vi "client.vi"() -> ()   [LabVIEW 2016]
uses:
  defs/Control 1.ctl
  defs/Control 3.ctl
  defs/Control 2.ctl
  defs/Control 6.ctl
  defs/Control 5.ctl
  defs/Control 4.ctl
panel:
  in  "czestotl [Hz]":T1=1.0
  in  "jaki sygna³?":T2 items=["sin", "square", "sawtooth", "noise"]
  in  "z jakim?":T3 items=["sin", "square", "sawtooth", "noise"]
  in  "dzialanie":T4 items=["+", "-", "*", "/", ""]
  in  "amplituda":T5=10.0 caption="Frequency"
  in  "x pocz":T1
  in  "Clear":bool
  out "wynik dzialania":cluster{"Y":dbl[], "Y":dbl[]}[](graph)
  in  "krok [ms]":T6=50.0 caption="Frequency"
  in  "Stop":bool
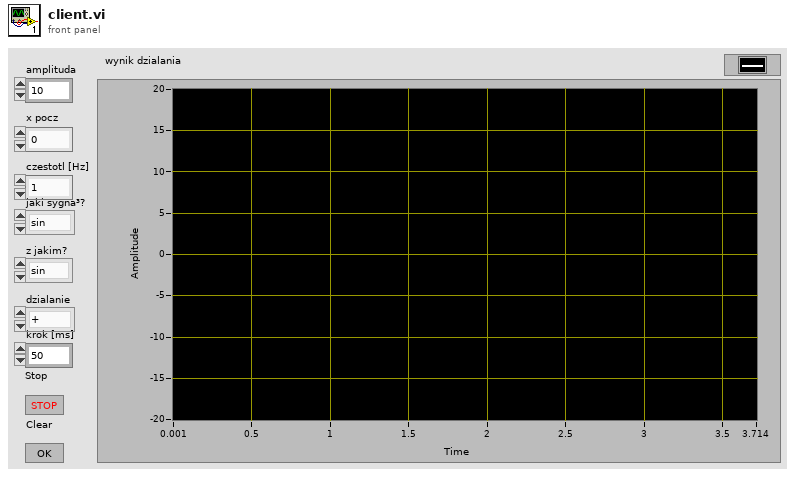
[diagram p1: front panel]
types:
  T1 = typedef "Control 3.ctl" = dbl
  T2 = typedef "Control 4.ctl" = u16
  T3 = typedef "Control 5.ctl" = u16
  T4 = typedef "Control 6.ctl" = u16
  T5 = typedef "Control 2.ctl" = dbl
  T6 = typedef "Control 1.ctl" = dbl
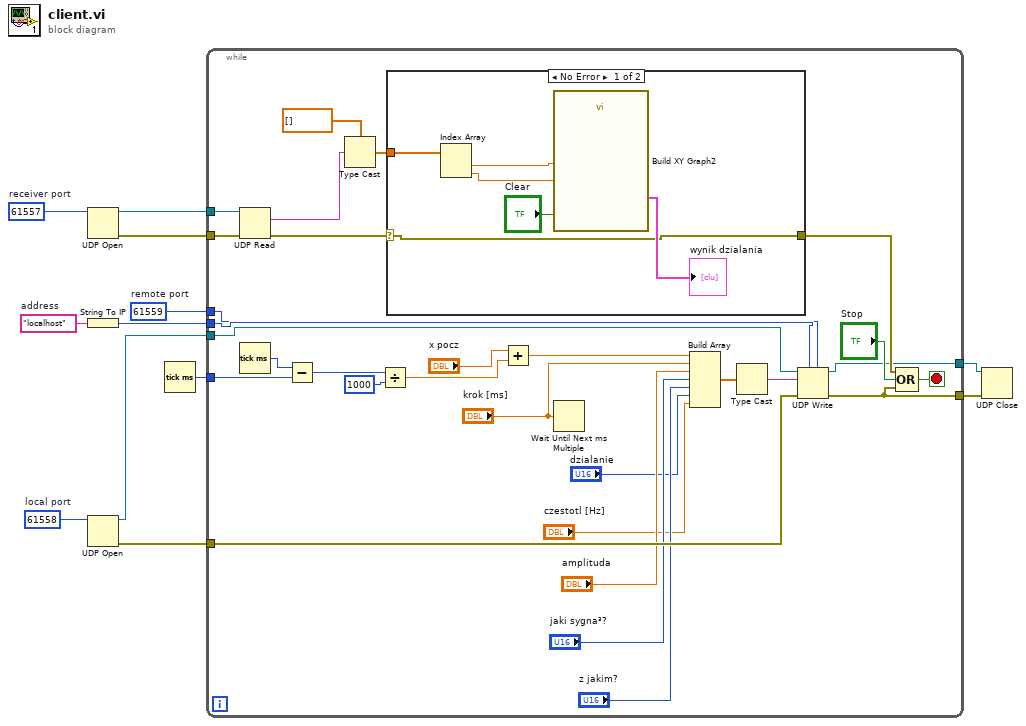
[diagram p0: block diagram]
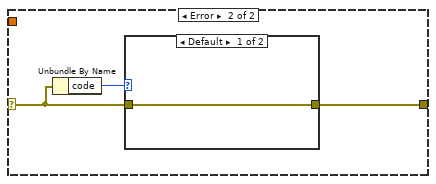
[diagram p2: hidden frame]
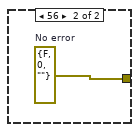
[diagram p3: hidden frame]
diagram:
  w3 = u16 61559  # remote port
  w8 = u16 61558  # local port
  w9 = "localhost"  # address
  w12 = u16 61557  # receiver port
  n1 = UDP Open(11:w12) -> (port=w11:refnum<k16>, 0:w10:errorcluster)  [unwired: 4 in, 1 out]
  n2 = String To IP(1:w9) -> (0:w6:u32)
  n3 = UDP Open(11:w8) -> (port=w4:refnum<k16>, 0:w5:errorcluster)  [unwired: 4 in, 1 out]
  n4 = Tick Count (ms)() -> (millisecond timer value=w7:u32)
  n5 = while {
    tunnel: w11 -> [w42]
    tunnel: w10 -> [w41]
    tunnel: w7 -> [w26]
    tunnel: w6 -> [w25]
    tunnel: w5 -> [w24]
    tunnel: w4 -> [w23]
    tunnel: w3 -> [w22]
    tunnel: [w21] -> w2
    tunnel: [w20] -> w1
    stop <- w34 stop-if-true
    n6 = UDP Read(connection ID=w42, 8:w41) -> (data out=w39:string, error out=w40:errorcluster)  [unwired: 1 in, 4 out]
    n7 = Tick Count (ms)() -> (millisecond timer value=w27:u32)
    n8 = Subtract(x=w27, y=w26) -> (x-y=w29:u32)
    n9 = Type Cast(type=dbl[] [], x=w39) -> (*(type *) &x=w38:dbl[])
    n10 = Divide(x=w29, y=1000) -> (x/y=w28:dbl)
    n11 = case shown="No Error" w40 {
      selector: w40 -> [w43 w49]
      tunnel: w38 -> [w44 _]
      tunnel: [w43 w50] -> w35
      frame No Error {
        n12 = Index Array(array=w44) -> (element #1=w46:dbl, element #2=w45:dbl)  [unwired: 2 in]
        n13 = call "Build XY Graph2"("Reset"="Clear", "Y Input"=w45, "X Input"=w46) -> ("XY Graph"=→"wynik dzialania":cluster{"Y":dbl[], "Y":dbl[]}[])  [unwired: 7 in, 1 out]
      }
      frame Error {
        n14 = Unbundle By Name(w49) -> ("code"=w51:i32)
        n15 = case shown="Default" w51 {
          tunnel: [w52 w53] -> w50
          tunnel: w49 -> [w52 _]
          frame Default {
          }
          frame 56 {
            w53 = errorcluster {"status"=FALSE, "code"=0, "source"=""}  # No error
          }
        }
      }
    }
    n16 = Add(x="x pocz", y=w28) -> (x+y=w13:T1)
    n17 = Wait Until Next ms Multiple(millisecond multiple="krok [ms]") -> ()  [unwired: 1 out]
    n18 = Build Array(w13, "krok [ms]", "amplituda", "jaki sygna³?", "z jakim?", "dzialanie", "czestotl [Hz]") -> (w31:T1[])
    n19 = Type Cast(x=w31) -> (*(type *) &x=w32:string)  [unwired: 1 out]
    n20 = UDP Write(address=w25, port or service name=w22, connection ID=w23, data in=w32, 8:w24) -> (error out=w20:errorcluster, 3:w21:refnum<k16>)  [unwired: 1 in]
    n21 = Compound Arithmetic op=OR(w35, "Stop", w20) -> (w34:bool)
  }
  n22 = UDP Close(connection ID=w2, 8:w1) -> ()  [unwired: 2 out]
